vi "TestVI.vi"() -> ()   [LabVIEW 2015, in "Schedule Modul.lvlib"]
uses:
  Schedule Modul.lvlib
panel:
  in  "Stopp":bool
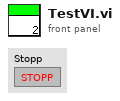
[diagram p1: front panel]
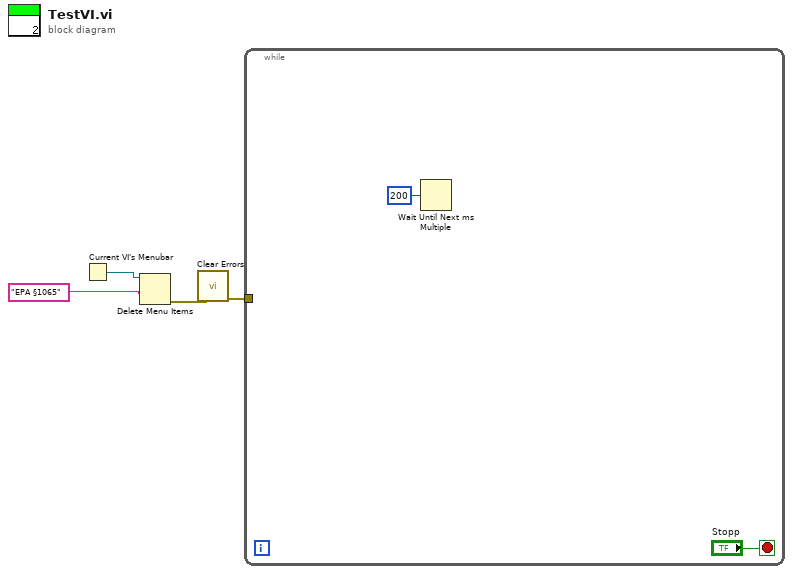
[diagram p0: block diagram]
diagram:
  n1 = Current VI's Menubar() -> (w2:refnum<k9>)
  n2 = Delete Menu Items(7:"EPA §1065" ("Menüpunkt-Tag"), 9:w2) -> (0:w4:errorcluster)  [unwired: 2 in, 1 out]
  n3 = call <vilib>:"Clear Errors.vi"("error in (no error)"=w4) -> ("error out"=w3:errorcluster)  [unwired: 5 in, 1 out]
  n4 = while {
    tunnel: w3 -> [_]
    stop <- "Stopp" stop-if-true
    n5 = Wait Until Next ms Multiple(millisecond multiple=u32 200 ("ms")) -> ()  [unwired: 1 out]
  }
